vi "Modbus Write U32.vi"(7 "Slave Address":u8, 8 "error in (no error)":errorcluster, 9 "Input data U32":u32, 10 "Register Start Address":u16 format="%x", 11 "VISA resource in":refnum<visa-resource-name>) -> (0 "error out":errorcluster, 3 "VISA resource out":refnum<visa-resource-name>)   [LabVIEW 2023, in "Voegtlin_NI_SMART_Modbus_Drivers.lvlib"]
doc: "Schreibe einen U32-Wert an die angegebene Startadresse des selektierten Geraetes.\nDer COM-Port muss dazu initialisiert sein (benutze\" Modbus Init.vi\")."
uses:
  Voegtlin_NI_SMART_Modbus_Drivers.lvlib
  Enums/Modbus Comm.ctl
panel:
  out "U16 input data to write\n(array)":u16[](array[numeric])
  # "Input Data"
  # "Internal Data"
  # "Output Data"
  # "(Inputmaske in HEX)"
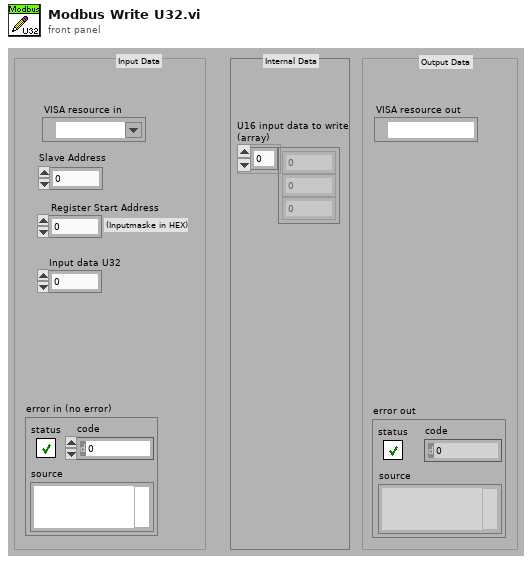
[diagram p1: front panel]
types:
  T1 = typedef "Voegtlin_NI_SMART_Modbus_Drivers.lvlib/Modbus Comm.ctl" = enum16{"Init", "Read", "Write", "Exit"}
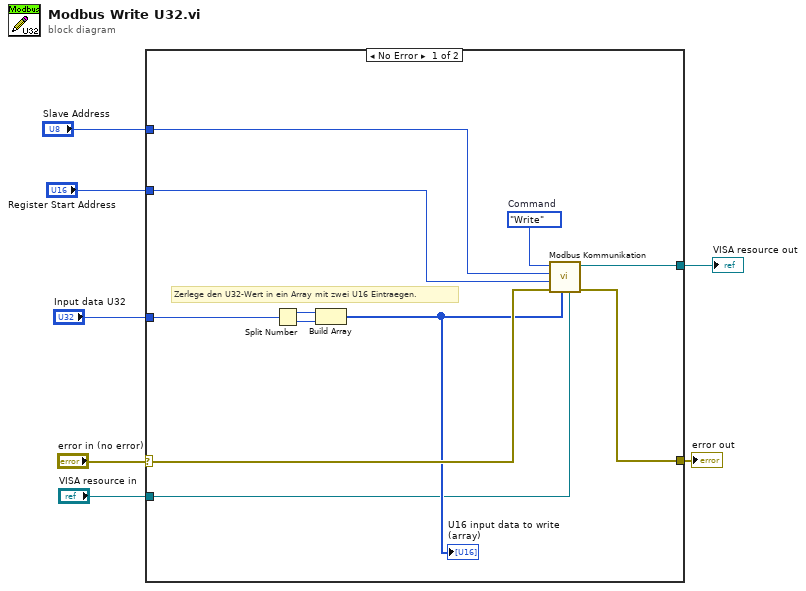
[diagram p0: block diagram]
diagram:
  n1 = case shown="No Error" "error in (no error)" {
    selector: "error in (no error)" -> [w13 w20]
    tunnel: [w17 w20] -> w7
    tunnel: "Register Start Address" -> [w11 _]
    tunnel: "Input data U32" -> [w14 _]
    tunnel: "Slave Address" -> [w10 _]
    tunnel: "VISA resource in" -> [w9 w19]
    tunnel: [w8 w19] -> w1
    frame No Error {
      w18 = Modbus_Comm."Write"  # Command
      # "Zerlege den U32-Wert in ein Array mit zwei U16 Eintraegen."
      n2 = Split Number(x=w14) -> (hi(x)=w16:u16, lo(x)=w15:u16)
      n3 = Build Array(w16, w15) -> (w12:u16[])
      "U16 input data to write\n(array)" <- w12
      n4 = call "Modbus Kommunikation.vi"("VISA resource in"=w9, "Data In / #Reads [U16]"=w12, "error in (no error)"=w13, "Register Start Address"=w11, "Slave Address"=w10, "Command"=w18) -> ("error out"=w17:errorcluster, "VISA resource out"=w8:refnum<visa-resource-name>)  [unwired: 3 in, 1 out]
    }
    frame Error {
    }
  }
  "error out" <- w7
  "VISA resource out" <- w1
